vi "Get Main Page Monitor Log Directory.vi"(8 "error in":errorcluster, 11 "Main Page Ref in":T1 format="%.0x") -> (0 "error out":errorcluster, 2 "Monitor Log Directory":string, 3 "Main Page Ref out":T1 format="%.0x", 4 "Found?":bool)   [LabVIEW 2020, in "AIM ARINC 664 Scripting.lvlib"]
uses:
  AIM ARINC 664 Scripting.lvlib
  <vilib>/NI VeriStand/Custom Device API/Custom Device API.lvlib
  Constants.vi
  <vilib>/NI VeriStand/Custom Device API/Get Item Property (String).vi
  <vilib>/NI VeriStand/Custom Device API/Custom Device Item Ref.ctl
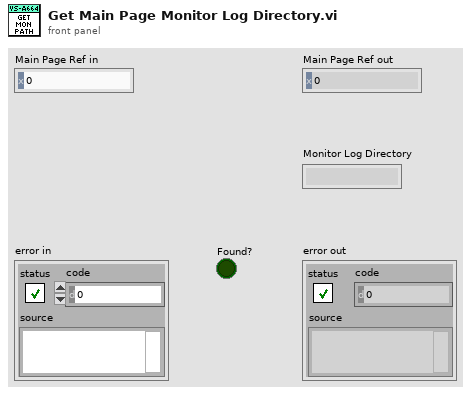
[diagram p1: front panel]
types:
  T1 = typedef "Custom Device API.lvlib/Custom Device Item Ref.ctl" = u64
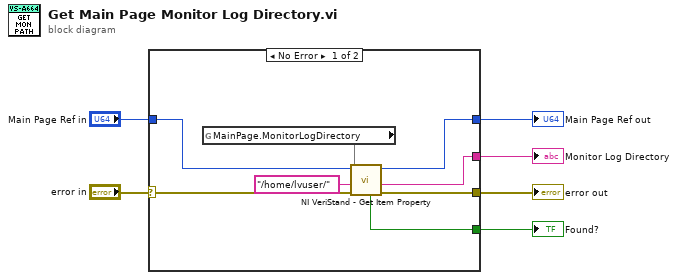
[diagram p0: block diagram]
diagram:
  n1 = case shown="No Error" "error in" {
    selector: "error in" -> [w8 w16]
    tunnel: "Main Page Ref in" -> [w12 w15]
    tunnel: [w14 w16] -> w5
    tunnel: [w13 w15] -> w4
    tunnel: [w11 _] -> w2
    tunnel: [w10 _] -> w1
    frame No Error {
      n2 = global read "Constants.vi" "MainPage.MonitorLogDirectory"() -> (w9)
      n3 = call-poly <vilib>:"NI VeriStand - Get Item Property.vi"("error in (no error)"=w8, "Default Value"="/home/lvuser/", "Property Name"=w9, "Item Ref in"=w12) -> ("error out"=w14:errorcluster, "Value"=w11:string, "Item Ref out"=w13:T1, "Found?"=w10:bool)  [unwired: 4 in]
    }
    frame Error {
    }
  }
  "error out" <- w5
  "Monitor Log Directory" <- w2
  "Main Page Ref out" <- w4
  "Found?" <- w1
